vi "例程51-动画设置指定VI中的控件属性.vi"() -> ()   [LabVIEW 2016]
panel:
  in  "控件名":string="幅值"
  in  "停止":bool
  in  "数值":dbl=0.02 format="%.2g"
  in  "VI路径":path=path "C:/Users/abao/Desktop/LabView例程/例程51-动态波形幅值.vi"
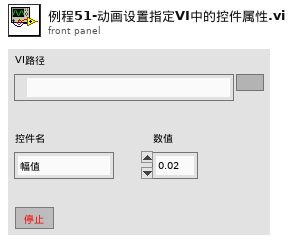
[diagram p1: front panel]
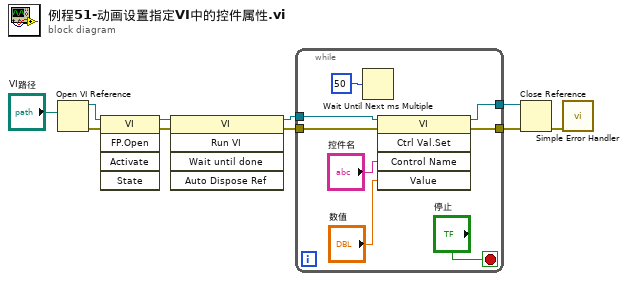
[diagram p0: block diagram]
diagram:
  n1 = Open VI Reference(vi path="VI路径") -> (vi reference=w9:refnum<vi>, error out=w8:errorcluster)  [unwired: 5 in]
  n2 = invoke class="VI" method="FP.Open"(reference=w9, error in=w8) -> (reference out=w4:refnum<vi>, error out=w3:errorcluster)  [unwired: 3 in, 3 out]
  n3 = invoke class="VI" method="Run VI"(reference=w4, error in=w3) -> (reference out=w2:refnum<vi>, error out=w1:errorcluster)  [unwired: 3 in, 3 out]
  n4 = while {
    tunnel: [w14] -> w7
    tunnel: [w13] -> w6
    tunnel: w2 -> [w12]
    tunnel: w1 -> [w11]
    stop <- "停止" stop-if-true
    n5 = Wait Until Next ms Multiple(millisecond multiple=u32 50 ("毫秒倍数")) -> ()  [unwired: 1 out]
    n6 = invoke class="VI" method="Ctrl Val.Set"(reference=w12, error in=w11, "Control Name"="控件名", "Value"="数值") -> (reference out=w14:refnum<vi>, error out=w13:errorcluster)  [unwired: 1 in, 3 out]
  }
  n7 = Close Reference(reference=w7, error in (no error)=w6) -> (error out=w5:errorcluster)
  n8 = call <vilib>:"Simple Error Handler.vi"("error in (no error)"=w5) -> ()  [unwired: 4 in, 5 out]
